vi "Flash读写实验.vi"() -> ()   [LabVIEW 2011]
uses:
  <vilib>/STM32_DriverVI_Interface_F4/SPI/SPI Comm Speed_F4.ctl
  <vilib>/STM32_DriverVI_Interface_F4/SPI/SPI2_SCK_Pin_Map_F4.ctl
  <vilib>/STM32_DriverVI_Interface_F4/SPI/SPI2_MISO_Pin_Map_F4.ctl
  <vilib>/STM32_DriverVI_Interface_F4/SPI/SPI2_MOSI_Pin_Map_F4.ctl
  <vilib>/STM32_DriverVI_Interface_F4/GPIO/GPI_Single_Interface_F4.ctl
  <vilib>/STM32_DriverVI_Interface_F4/LCD/Show_Mode_F4.ctl
  <vilib>/STM32_DriverVI_Interface_F4/LCD/Font_Size_F4.ctl
  <vilib>/STM32_DriverVI_Interface_F4/LCD/Brush Color_Index_F4.ctl
  <vilib>/eio/EIO_TerminalDirection.ctl
  <vilib>/STM32_DriverVI_Interface_F4/LCD/LCD_Init_F4.vi
  <vilib>/STM32_DriverVI_Interface_F4/SPI/SPI2 Init_F4.vi
  <vilib>/STM32_DriverVI_Interface_F4/Flash-VI/SPI2 Flash ID Read_F4.vi
  <vilib>/STM32_DriverVI_Interface_F4/GPIO_EIO/GPI_EIO_Inner_F4.vi
  <vilib>/STM32_DriverVI_Interface_F4/Flash-C/SPI2 Flash Write-C_F4.vi
  <vilib>/STM32_DriverVI_Interface_F4/Flash-C/SPI2 Flash Read-C_F4.vi
  <vilib>/eio/EIONode/EIONode.xnode
panel:
  in  "Read Num Bytes":u16
  in  "x":bool
  out "字符串":string
  out "Flash_ID":string
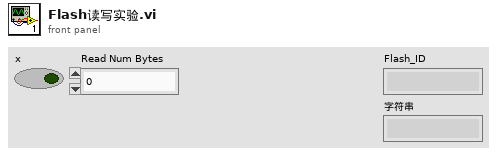
[diagram p1: front panel]
types:
  T1 = typedef "GPI_Single_Interface_F4.ctl" = enum8{"Port A.0", "Port A.1", "Port A.2", "Port A.3", "Port A.4", "Port A.5", "Port A.6", "Port A.7", "Port A.8", "Port A.9", "Port A.10", "Port A.11", "Port A.12", "Port A.13", "Port A.14", "Port A.15", "Port B.0", "Port B.1", "Port B.2", "Port B.3", "Port B.4", "Port B.5", "Port B.6", "Port B.7", "Port B.8", "Port B.9", "Port B.10", "Port B.11", "Port B.12", "Port B.13", "Port B.14", "Port B.15", "Port C.0", "Port C.1", "Port C.2", "Port C.3", "Port C.4", "Port C.5", "Port C.6", "Port C.7", "Port C.8", "Port C.9", "Port C.10", "Port C.11", "Port C.12", "Port C.13", "Port C.14", "Port C.15", "Port D.0", "Port D.1", "Port D.2", "Port D.3", "Port D.4", "Port D.5", "Port D.6", "Port D.7", "Port D.8", "Port D.9", "Port D.10", "Port D.11", "Port D.12", "Port D.13", "Port D.14", "Port D.15", "Port E.0", "Port E.1", "Port E.2", "Port E.3", "Port E.4", "Port E.5", "Port E.6", "Port E.7", "Port E.8", "Port E.9", "Port E.10", "Port E.11", "Port E.12", "Port E.13", "Port E.14", "Port E.15", "Port F.0", "Port F.1", "Port F.2", "Port F.3", "Port F.4", "Port F.5", "Port F.6", "Port F.7", "Port F.8", "Port F.9", "Port F.10", "Port F.11", "Port F.12", "Port F.13", "Port F.14", "Port F.15", "Port G.0", "Port G.1", "Port G.2", "Port G.3", "Port G.4", "Port G.5", "Port G.6", "Port G.7", "Port G.8", "Port G.9", "Port G.10", "Port G.11", "Port G.12", "Port G.13", "Port G.14", "Port G.15", "Port H.0", "Port H.1", "Port H.2", "Port H.3", "Port H.4", "Port H.5", "Port H.6", "Port H.7", "Port H.8", "Port H.9", "Port H.10", "Port H.11", "Port H.12", "Port H.13", "Port H.14", "Port H.15", "Port I.0", "Port I.1", "Port I.2", "Port I.3", "Port I.4", "Port I.5", "Port I.6", "Port I.7", "Port I.8", "Port I.9", "Port I.10", "Port I.11", "Port I.12", "Port I.13", "Port I.14", "Port I.15"}
  T2 = typedef "SPI2_MOSI_Pin_Map_F4.ctl" = u8
  T3 = typedef "SPI2_MISO_Pin_Map_F4.ctl" = u8
  T4 = typedef "SPI2_SCK_Pin_Map_F4.ctl" = u8
  T5 = typedef "SPI Comm Speed_F4.ctl" = enum8{"42.00  MHz", "21.00  MHz", "10.50  MHz", "5.250  MHz", "2.625  MHz", "1.3125MHz", "656.25kHz", "328.125kHz"}
  T6 = typedef "Show_Mode_F4.ctl" = enum8{"非叠加显示", "叠加显示"}
  T7 = typedef "Font_Size_F4.ctl" = enum8{"Small_Font（12）", "Big_Font（16）"}
  T8 = typedef "Brush Color_Index_F4.ctl" = enum8{"White", "Black", "Blue", "Green_Blue", "Red", "Magenta（品红）", "Green", "Cyan（青色）", "Yellow", "Brown", "Brown_Red", "Gray", "Dark_Blue", "Light_Blue", "Gray_Blue", "Light_Green", "Light_Gray", "Light_Gray_Blue", "Light_Brown_Blue"}
  T9 = enum8{"P0", "P1", "P2", "P3", "P4", "P5", "P6", "P7", "P8", "P9", "P10", "P11", "P12", "P13", "P14", "P15"}
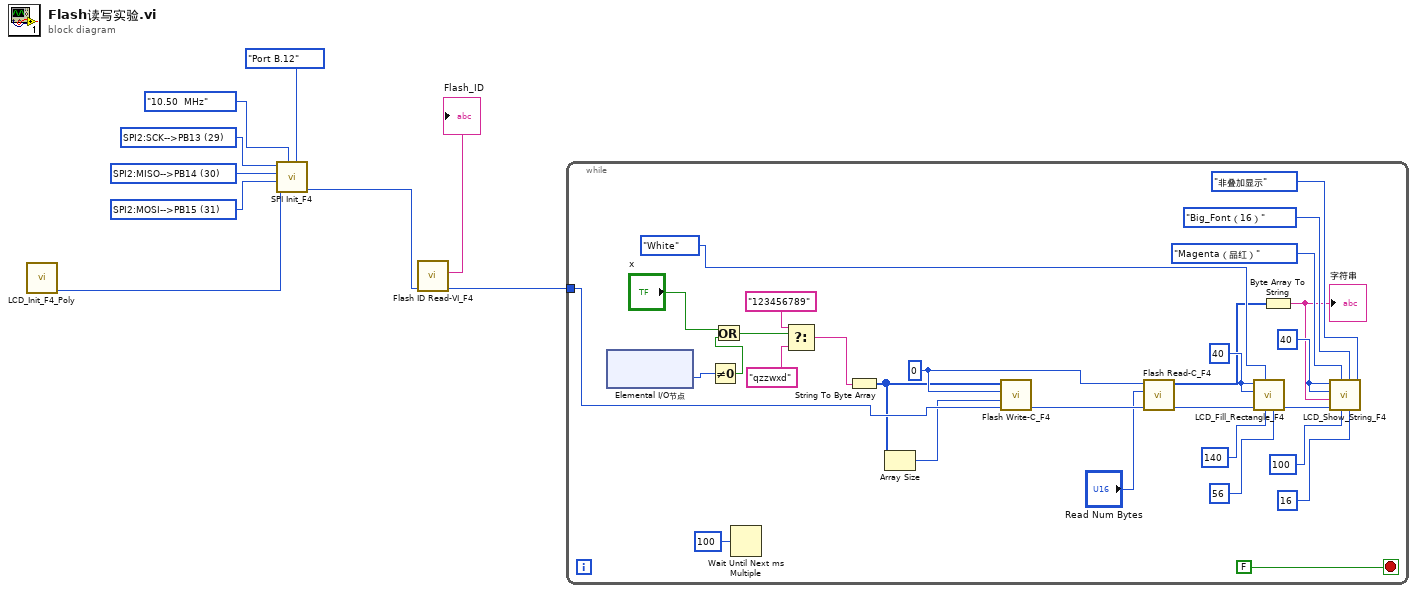
[diagram p0: block diagram]
diagram:
  w2 = T2 31 items=["SPI2:MOSI-->PB15"=31, "SPI2:MOSI-->PC3"=35, "SPI2:MOSI-->PI3"=131] ("SPI2_MOSI_Pin_Map")
  w3 = T3 30 items=["SPI2:MISO-->PB14"=30, "SPI2:MISO-->PC2"=34, "SPI2:MISO-->PI2"=130] ("SPI2_MISO_Pin_Map")
  w4 = T4 29 items=["SPI2:SCK-->PB10"=26, "SPI2:SCK-->PB13"=29, "SPI2:SCK-->PI1"=129] ("SPI2_SCK_Pin_Map")
  n1 = call-poly <vilib>:"LCD_Init_F4_Poly.vi"() -> ("err_out"=w9:u8)  [unwired: 10 in, 1 out]
  n2 = call-poly <vilib>:"SPI Init_F4.vi"("SPI2_NSS（CS）"=GPI_Single_Interface_F4."Port B.12", "SPI Comm Speed"=SPI_Comm_Speed_F4."10.50  MHz", "err_in"=w9, "SPI2_MOSI_Pin_Map"=w2, "SPI2_MISO_Pin_Map"=w3, "SPI2_SCK_Pin_Map"=w4) -> ("err_out"=w8:u8)  [unwired: 5 in]
  n3 = call-poly <vilib>:"Flash ID Read-VI_F4.vi"("err_in"=w8) -> ("err_out"=w5:u8, "Flash_ID"=→"Flash_ID":string)  [unwired: 8 in, 1 out]
  n4 = while {
    tunnel: w5 -> [w21]
    stop <- FALSE stop-if-true
    w33 = u16 40 ("X_Position")
    w37 = u16 40 ("X1_Position")
    w20 = u32 0 ("Address")
    n5 = xnode "Elemental I/O节点"() -> ("KEY_UP"=w17:u8)  [unwired: 1 in, 1 out]
    n6 = Not Equal To 0?(x=w17) -> (x != 0?=w15:bool)
    n7 = Or(x="x", y=w15) -> (x .or. y?=w14:bool)
    n8 = Wait Until Next ms Multiple(millisecond multiple=u32 100 ("毫秒倍数")) -> ()  [unwired: 1 out]
    n9 = Select(t="123456789", s=w14, f="qzzwxd") -> (s? t:f=w13:string)
    n10 = String To Byte Array(string=w13) -> (unsigned byte array=w19:u8[])
    n11 = Array Size(array=w19) -> (size(s)=w18:i32)
    n12 = call-poly <vilib>:"Flash Write-C_F4.vi"("err_in"=w21, "Length"=w18, "Address"=w20, "Write Data[U8]"=w19) -> ("err_out"=w22:u8)  [unwired: 7 in]
    n13 = call-poly <vilib>:"Flash Read-C_F4.vi"("err_in"=w22, "Read Num Bytes"="Read Num Bytes", "Address"=w20) -> ("err_out"=w24:u8, "Read Data[U8]"=w25:u8[])  [unwired: 7 in]
    n14 = call <vilib>:"LCD_Fill_Rectangle_F4.vi"("Y2_Position"=u16 56, "X2_Position"=u16 140, "Brush Color"=Brush_Color_Index_F4."White", "err_in"=w24, "Y1_Position"=w37, "X1_Position"=w37) -> ("err_out"=w34:u8)  [unwired: 5 in]
    n15 = Byte Array To String(unsigned byte array=w25) -> (string=w23:string)
    "字符串" <- w23
    n16 = call <vilib>:"LCD_Show_String_F4.vi"("Show_Mode"=Show_Mode_F4."非叠加显示", "Height"=u16 16, "Font_Size"=Font_Size_F4."Big_Font（16）", "Width"=u16 100, "Brush Color"=Brush_Color_Index_F4."Magenta（品红）", "err_in"=w34, "String"=w23, "Y_Position"=w33, "X_Position"=w33) -> ()  [unwired: 2 in, 1 out]
  }
